vi "Inline Rx Wait.vi"(8 "error in (no error)":errorcluster, 10 "Dispatcher Interface in":refnum<class "Dispatcher Interface.lvclass">, 11 "Plugin Timing Group in":refnum<class "Plugin Timing Group.lvclass">) -> (0 "error out":errorcluster, 2 "Dispatcher Interface out":refnum<class "Dispatcher Interface.lvclass">, 3 "Plugin Timing Group out":refnum<class "Plugin Timing Group.lvclass">)   [LabVIEW 2017, in "DSF Core.lvlib" / "Plugin Timing Group.lvclass"]
uses:
  Timing/Plugin Timing Group.lvclass
  Interfaces/Dispatcher/Dispatcher Interface.lvclass
  Timing/Transfer Group Timing.lvclass
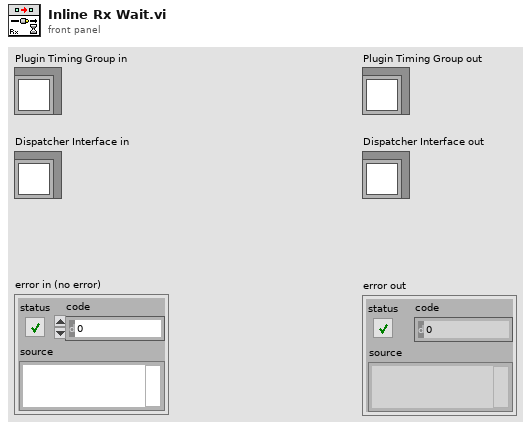
[diagram p1: front panel]
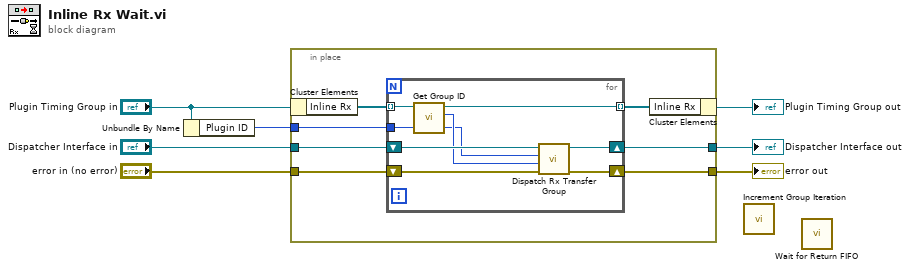
[diagram p0: block diagram]
diagram:
  n1 = Unbundle By Name("Plugin Timing Group in") -> ("Plugin ID"=w1:i32)
  n2 = in-place {
    in-place-border: "Dispatcher Interface in" -> [w12]
    in-place-border: [w11] -> w5
    in-place-border: [w10] -> w3
    in-place-border: "error in (no error)" -> [w9]
    in-place-border: w1 -> [w8]
    n3 = in-place-cluster #1("Plugin Timing Group in") -> ("Inline Rx"=w14:refnum<class "Transfer Group Timing.lvclass">[])
    n4 = for {
      tunnel: w14 -> [w18] mode=indexing
      tunnel: [w17] -> w13 mode=indexing
      shift-right: [w21] -> w11
      shift-left: w12 -> [w22]
      shift-right: [w20] -> w10
      shift-left: w9 -> [w19]
      tunnel: w8 -> [w15]
      n5 = call "Get Group ID.vi"("Transfer Group Timing in"=w18) -> ("Group ID"=w16:i32, "Transfer Group Timing out"=w17:refnum<class "Transfer Group Timing.lvclass">)  [unwired: 9 in]
      n6 = call "Dispatch Rx Transfer Group.vi"("error in (no error)"=w19, "Transfer Group ID"=w16, "Plugin ID"=w15, "Dispatcher Interface in"=w22) -> ("error out"=w20:errorcluster, "Dispatcher Interface out"=w21:refnum<class "Dispatcher Interface.lvclass">)  [unwired: 6 in]
    }
    n7 = in-place-cluster #1("Inline Rx"=w13) -> (→"Plugin Timing Group out":refnum<class "Plugin Timing Group.lvclass">)
  }
  "Dispatcher Interface out" <- w5
  "error out" <- w3
  n8 = call "Increment Group Iteration.vi"() -> ()  [unwired: 10 in, 2 out]
  n9 = call "Wait for Return FIFO.vi"() -> ()  [unwired: 9 in, 3 out]
